vi "PM100D2&D3 SCPI Example.vi"() -> ()   [LabVIEW 2015]
uses:
  <vilib>/ErrorRing/Error Ring.xnode
  <vilib>/Utility/error.llb/Error Cluster From Error Code.vi
panel:
  in  "stop":bool
  out "ARR LEN":i32
  out "rate":dbl format="%#.2f"
  out "count":i32
  out "time":u32
  out "error out":errorcluster
  in  "Tab Control":T1(tab)
  out "Chart":dbl(graph)
  in  "Scope Mode Array Length":i32=100
  out "Scope Mode Array [timestamp(us), power(W)]":cluster{u32, sgl}[](array[cluster])
  in  "Burst Mode Array Length":i32=100
  out "Burst Mode Array [timestamp(us), power(W)]":cluster{u32, sgl}[](array[cluster])
  out "Product Info":string
  # "Average Sampling Rate (Samples/s)"
  # "(range is 1 to 100)"
  # "I/O ports are 5 V TTL tolerant. The start of measurement is triggered on the rising edge of the TTL signal. In this example, the GPIO1 is configured as IALT."
  # "(range is 1 to 100)"
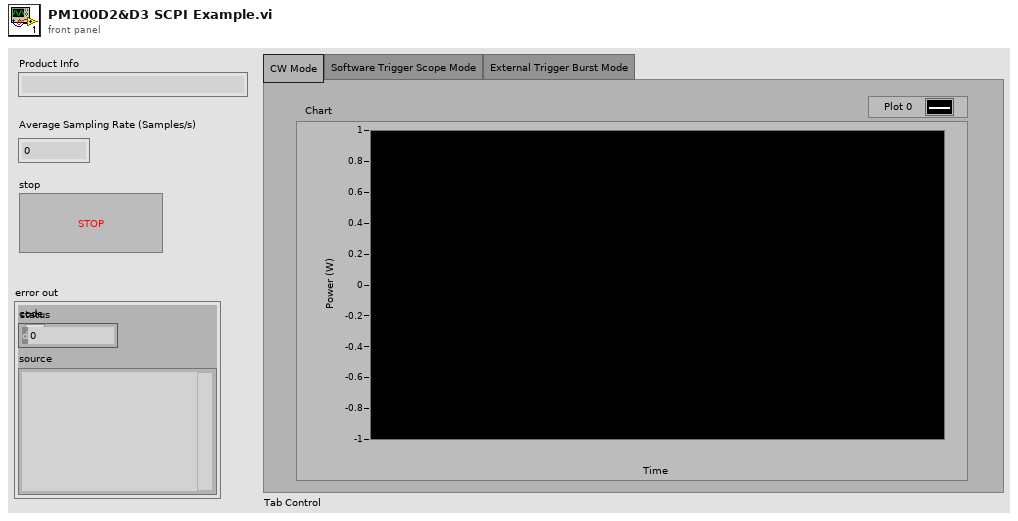
[diagram p1: front panel]
types:
  T1 = enum32{"CW Mode", "Software Trigger Scope Mode", "External Trigger Burst Mode"}
  T2 = enum16{"big-endian, network order", "native, host order", "little-endian"}
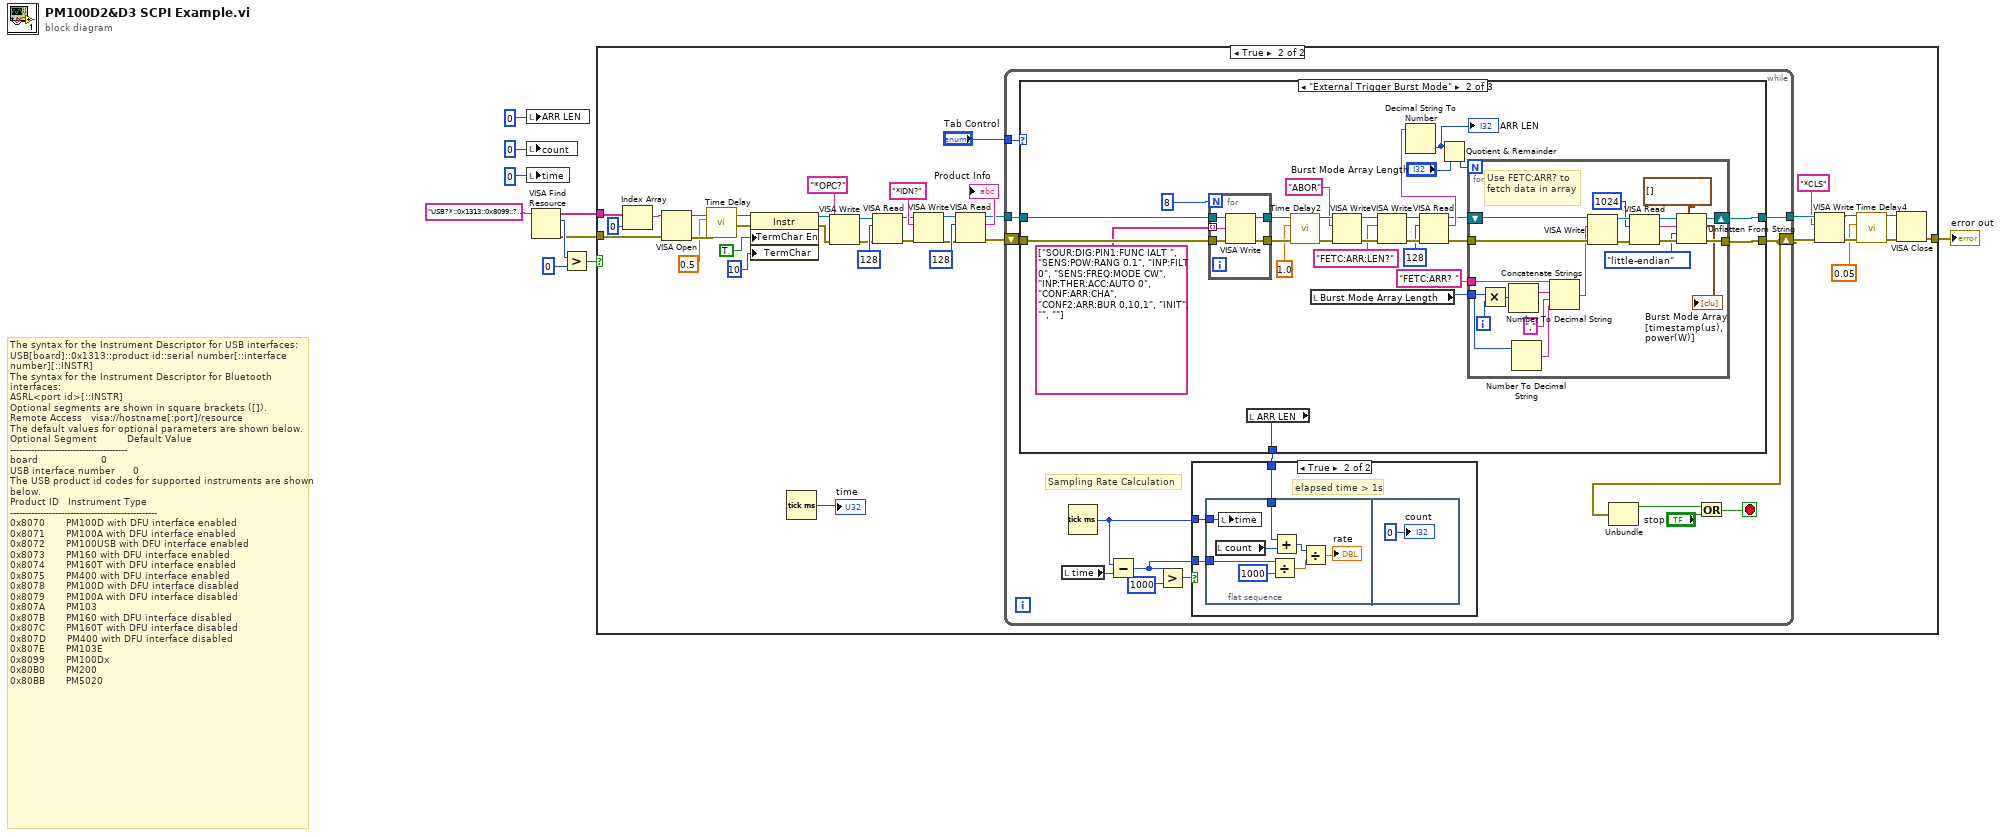
[diagram p0: block diagram]
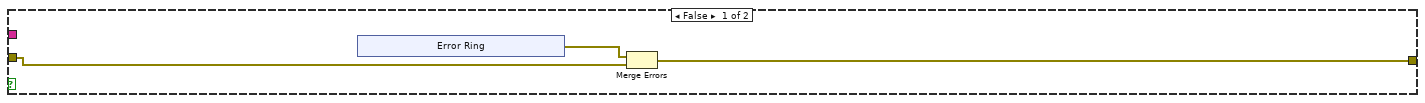
[diagram p2: hidden frame]
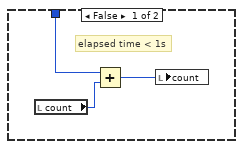
[diagram p3: hidden frame]
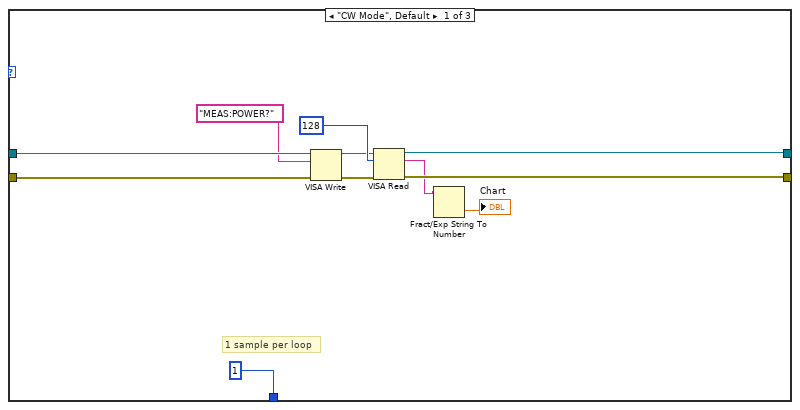
[diagram p4: hidden frame]
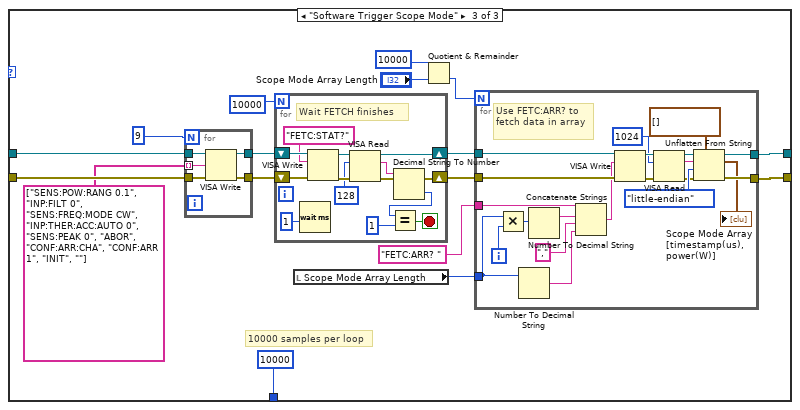
[diagram p5: hidden frame]
diagram:
  # "The syntax for the Instrument Descriptor for USB interfaces:\nUSB[board]::0x1313::product id::serial number[::interface number][::INSTR]\nThe syntax for the Instrument Descriptor for Bluetooth interfaces:\nASRL<port id>[::INSTR]\nOptional segments are shown in square brackets ([]).\nRemote Access   visa://hostname[:port]/resource\nThe default values for optional parameters are shown below.\nOptional Segment          Default Value\n---------------------------------------\nboard                     0\nUSB interface number      0\nThe USB product id codes for supported instruments are shown below.\nProduct ID   Instrument Type\n-------------------------------------------------\n0x8070       PM100D with DFU interface enabled\n0x8071       PM100A with DFU interface enabled\n0x8072       PM100USB with DFU interface enabled\n0x8073       PM160 with DFU interface enabled\n0x8074       PM160T with DFU interface enabled\n0x8075       PM400 with DFU interface enabled\n0x8078       PM100D with DFU interface disabled\n0x8079       PM100A with DFU interface disabled\n0x807A       PM103\n0x807B       PM160 with DFU interface disabled\n0x807C       PM160T with DFU interface disabled\n0x807D       PM400 with DFU interface disabled\n0x807E       PM103E\n0x8099       PM100Dx\n0x80B0       PM200\n0x80BB       PM5020"
  n1 = local write "ARR LEN"(0 ("ARR LEN")) -> ()
  n2 = local write "count"(0 ("loopCount")) -> ()
  n3 = local write "time"(u32 0 ("time")) -> ()
  n4 = VISA Find Resource(11:"USB?*::0x1313::0x8099::?*::INSTR" ("expression (\"?*\")")) -> (0:w4:errorcluster, 2:w9:u32, 3:w6:string[])  [unwired: 2 in]
  n5 = Greater?(x=w9, y=u32 0) -> (0:w7:bool)
  n6 = case shown="True" w7 {
    tunnel: w6 -> [_ w53]
    tunnel: [w13 w26] -> w5
    tunnel: w4 -> [w12 w38]
    frame False {
      n7 = xnode "Error Ring"() -> ("error out"=w11:errorcluster)
      n8 = Merge Errors(w11, w12) -> (w13:errorcluster)
    }
    frame True {
      n9 = Index Array(array=w53, index=0) -> (element=w39:string)
      n10 = VISA Open(error in (no error)=w38, VISA resource name=w39) -> (VISA resource name=w45:refnum<visa-resource-name>, error out=w48:errorcluster)  [unwired: 3 in]
      n11 = call "Time Delay"("error in (no error)"=w48, "Delay Time (s)"=0.5) -> ("error out"=w46:errorcluster)  [unwired: 9 in]
      n12 = property class="Instr"(reference=w45, error in=w46, "TermChar En"=TRUE ("Message Based Settings:Termination Character Enable"), "TermChar"=u8 10 ("Message Based Settings:Termination Character")) -> (reference out=w22:refnum<visa-resource-name>, error out=w21:errorcluster)
      n13 = Tick Count (ms)() -> (millisecond timer value=→"time":u32)
      n14 = VISA Write(VISA resource name=w22, write buffer="*OPC?", error in (no error)=w21) -> (VISA resource name out=w34:refnum<visa-resource-name>, error out=w19:errorcluster)  [unwired: 1 out]
      n15 = VISA Read(VISA resource name=w34, byte count=u32 128, error in (no error)=w19) -> (VISA resource name out=w33:refnum<visa-resource-name>, error out=w36:errorcluster)  [unwired: 2 out]
      n16 = VISA Write(VISA resource name=w33, write buffer="*IDN?", error in (no error)=w36) -> (VISA resource name out=w50:refnum<visa-resource-name>, error out=w25:errorcluster)  [unwired: 1 out]
      n17 = VISA Read(VISA resource name=w50, byte count=u32 128, error in (no error)=w25) -> (VISA resource name out=w42:refnum<visa-resource-name>, read buffer=→"Product Info":string, error out=w41:errorcluster)  [unwired: 1 out]
      n18 = while {
        tunnel: [w67] -> w31
        tunnel: w42 -> [w66]
        tunnel: "Tab Control" -> [w64]
        shift-right: [w56] -> w32
        shift-left: w41 -> [w65]
        stop <- w54 stop-if-true
        # "Sampling Rate Calculation"
        n19 = case shown="\"External Trigger Burst Mode\"" w64 {
          tunnel: [w90 w117 w159] -> w67
          tunnel: w66 -> [w92 w118 w160]
          tunnel: [w89 w119 w161] -> w56
          tunnel: w65 -> [w91 w116 w146]
          tunnel: [1 w115 10000 ("x")] -> w61
          frame "CW Mode", Default {
            # "1 sample per loop"
            n20 = VISA Write(VISA resource name=w92, write buffer="MEAS:POWER?", error in (no error)=w91) -> (VISA resource name out=w84:refnum<visa-resource-name>, error out=w83:errorcluster)  [unwired: 1 out]
            n21 = VISA Read(VISA resource name=w84, byte count=u32 128, error in (no error)=w83) -> (VISA resource name out=w90:refnum<visa-resource-name>, read buffer=w87:string, error out=w89:errorcluster)  [unwired: 1 out]
            n22 = Fract/Exp String To Number(string=w87) -> (number=→"Chart":dbl)  [unwired: 3 in, 1 out]
          }
          frame "External Trigger Burst Mode" {
            n23 = for {
              N: 8 -> [_]
              tunnel: string[] ["SOUR:DIG:PIN1:FUNC IALT ", "SENS:POW:RANG 0.1", "INP:FILT 0", "SENS:FREQ:MODE CW", "INP:THER:ACC:AUTO 0", "CONF:ARR:CHA", "CONF2:ARR:BUR 0,10,1", "INIT", "", ""] -> [w142] mode=indexing
              tunnel: w116 -> [w144]
              tunnel: w118 -> [w143]
              tunnel: [w141] -> w112
              tunnel: [w140] -> w109
              n24 = VISA Write(VISA resource name=w143, write buffer=w142, error in (no error)=w144) -> (VISA resource name out=w140:refnum<visa-resource-name>, error out=w141:errorcluster)  [unwired: 1 out]
            }
            n25 = local read "ARR LEN"() -> (w115:i32)
            n26 = call "Time Delay2"("error in (no error)"=w112, "Delay Time (s)"=1.0) -> ("error out"=w110:errorcluster)  [unwired: 9 in]
            n27 = local read "Burst Mode Array Length"() -> (w94:i32)
            n28 = VISA Write(VISA resource name=w109, write buffer="ABOR", error in (no error)=w110) -> (VISA resource name out=w106:refnum<visa-resource-name>, error out=w107:errorcluster)  [unwired: 1 out]
            n29 = VISA Write(VISA resource name=w106, write buffer="FETC:ARR:LEN?", error in (no error)=w107) -> (VISA resource name out=w103:refnum<visa-resource-name>, error out=w104:errorcluster)  [unwired: 1 out]
            n30 = VISA Read(VISA resource name=w103, byte count=u32 128, error in (no error)=w104) -> (VISA resource name out=w99:refnum<visa-resource-name>, read buffer=w101:string, error out=w100:errorcluster)  [unwired: 1 out]
            n31 = Decimal String To Number(string=w101) -> (number=w97:i32)  [unwired: 2 in, 1 out]
            "ARR LEN" <- w97
            n32 = Quotient & Remainder(x=w97, y="Burst Mode Array Length") -> (floor(x/y)=w95:i32)  [unwired: 1 out]
            n33 = for {
              N: w95 -> [_]
              tunnel: w100 -> [w139]
              tunnel: "FETC:ARR? " ("write buffer") -> [w129]
              tunnel: [w126] -> w119
              tunnel: w94 -> [w121]
              shift-right: [w134] -> w117
              shift-left: w99 -> [w137]
              i -> [w120]
              # "Use FETC:ARR? to fetch data in array"
              n34 = Multiply(x=w121, y=w120) -> (x*y=w131:i32)
              n35 = Number To Decimal String(number=w131) -> (decimal integer string=w133:string)  [unwired: 1 in]
              n36 = Number To Decimal String(number=w121) -> (decimal integer string=w130:string)  [unwired: 1 in]
              n37 = Concatenate Strings(w129, w133, "," ("string"), w130) -> (w128:string)
              n38 = VISA Write(VISA resource name=w137, write buffer=w128, error in (no error)=w139) -> (VISA resource name out=w136:refnum<visa-resource-name>, error out=w138:errorcluster)  [unwired: 1 out]
              n39 = VISA Read(VISA resource name=w136, byte count=u32 1024, error in (no error)=w138) -> (VISA resource name out=w134:refnum<visa-resource-name>, read buffer=w123:string, error out=w127:errorcluster)  [unwired: 1 out]
              n40 = Unflatten From String(type=cluster{u32, sgl}[] [], binary string=w123, byte order (0:big-endian, network order)=T2."little-endian", error in (no error)=w127) -> (value=→"Burst Mode Array [timestamp(us), power(W)]":cluster{u32, sgl}[], error out=w126:errorcluster)  [unwired: 1 in, 1 out]
            }
          }
          frame "Software Trigger Scope Mode" {
            # "10000 samples per loop"
            n41 = for {
              N: 9 -> [_]
              tunnel: w146 -> [w199]
              tunnel: w160 -> [w198]
              tunnel: [w197] -> w152
              tunnel: [w196] -> w156
              tunnel: string[] ["SENS:POW:RANG 0.1", "INP:FILT 0", "SENS:FREQ:MODE CW", "INP:THER:ACC:AUTO 0", "SENS:PEAK 0", "ABOR", "CONF:ARR:CHA", "CONF:ARR 1", "INIT", ""] -> [w195] mode=indexing
              n42 = VISA Write(VISA resource name=w198, write buffer=w195, error in (no error)=w199) -> (VISA resource name out=w196:refnum<visa-resource-name>, error out=w197:errorcluster)  [unwired: 1 out]
            }
            n43 = for {
              N: 10000 -> [_]
              shift-right: [w169] -> w154
              shift-left: w156 -> [w174]
              shift-right: [w168] -> w153
              shift-left: w152 -> [w172]
              stop <- w163 stop-if-true
              # "Wait FETCH finishes"
              n44 = Wait (ms)(milliseconds to wait=u32 1) -> ()  [unwired: 1 out]
              n45 = VISA Write(VISA resource name=w174, write buffer="FETC:STAT?", error in (no error)=w172) -> (VISA resource name out=w170:refnum<visa-resource-name>, error out=w171:errorcluster)  [unwired: 1 out]
              n46 = VISA Read(VISA resource name=w170, byte count=u32 128, error in (no error)=w171) -> (VISA resource name out=w169:refnum<visa-resource-name>, read buffer=w166:string, error out=w168:errorcluster)  [unwired: 1 out]
              n47 = Decimal String To Number(string=w166) -> (number=w165:i32)  [unwired: 2 in, 1 out]
              n48 = Equal?(x=w165, y=1) -> (x = y?=w163:bool)
            }
            n49 = local read "Scope Mode Array Length"() -> (w147:i32)
            n50 = Quotient & Remainder(x=10000, y="Scope Mode Array Length") -> (floor(x/y)=w150:i32)  [unwired: 1 out]
            n51 = for {
              N: w150 -> [_]
              tunnel: w153 -> [w194]
              tunnel: w154 -> [w192]
              tunnel: "FETC:ARR? " ("write buffer") -> [w190]
              tunnel: [w186] -> w159
              tunnel: [w181] -> w161
              tunnel: w147 -> [w177]
              i -> [w179]
              # "Use FETC:ARR? to fetch data in array"
              n52 = Multiply(x=w177, y=w179) -> (x*y=w180:i32)
              n53 = Number To Decimal String(number=w177) -> (decimal integer string=w178:string)  [unwired: 1 in]
              n54 = Number To Decimal String(number=w180) -> (decimal integer string=w189:string)  [unwired: 1 in]
              n55 = Concatenate Strings(w190, w189, "," ("string"), w178) -> (w188:string)
              n56 = VISA Write(VISA resource name=w192, write buffer=w188, error in (no error)=w194) -> (VISA resource name out=w191:refnum<visa-resource-name>, error out=w193:errorcluster)  [unwired: 1 out]
              n57 = VISA Read(VISA resource name=w191, byte count=u32 1024, error in (no error)=w193) -> (VISA resource name out=w186:refnum<visa-resource-name>, read buffer=w184:string, error out=w182:errorcluster)  [unwired: 1 out]
              n58 = Unflatten From String(type=cluster{u32, sgl}[] [], binary string=w184, byte order (0:big-endian, network order)=T2."little-endian", error in (no error)=w182) -> (value=→"Scope Mode Array [timestamp(us), power(W)]":cluster{u32, sgl}[], error out=w181:errorcluster)  [unwired: 1 in, 1 out]
            }
          }
        }
        n59 = local read "time"() -> (w60:u32)
        n60 = Tick Count (ms)() -> (millisecond timer value=w62:u32)
        n61 = Subtract(x=w62, y=w60) -> (x-y=w59:u32)
        n62 = Greater?(x=w59, y=u32 1000) -> (0:w55:bool)
        n63 = case shown="True" w55 {
          tunnel: w62 -> [_ w73]
          tunnel: w61 -> [w69 w71]
          tunnel: w59 -> [_ w72]
          frame False {
            # "elapsed time < 1s"
            n64 = local read "count"() -> (w70:i32)
            n65 = Add(x=w69, y=w70) -> (x+y=w68:i32)
            n66 = local write "count"(w68) -> ()
          }
          frame True {
            # "elapsed time > 1s"
            n67 = flat-sequence {
              tunnel: w73 -> [w81]
              tunnel: w72 -> [w78]
              tunnel: w71 -> [w74]
              frame #0 {
                n68 = local read "count"() -> (w75:i32)
                n69 = local write "time"(w81) -> ()
                n70 = Divide(x=w78, y=u32 1000) -> (x/y=w79:dbl)
                n71 = Add(x=w74, y=w75) -> (x+y=w76:i32)
                n72 = Divide(x=w76, y=w79) -> (x/y=→"rate":dbl)
              }
              frame #1 {
                "count" <- 0 ("count")
              }
            }
          }
        }
        n73 = Unbundle(w56) -> ("status"=w57:bool)  [unwired: 2 out]
        n74 = Or(x=w57, y="stop") -> (x .or. y?=w54:bool)
      }
      n75 = VISA Write(VISA resource name=w31, write buffer="*CLS", error in (no error)=w32) -> (VISA resource name out=w30:refnum<visa-resource-name>, error out=w28:errorcluster)  [unwired: 1 out]
      n76 = call "Time Delay4"("error in (no error)"=w28, "Delay Time (s)"=0.05) -> ("error out"=w27:errorcluster)  [unwired: 9 in]
      n77 = VISA Close(VISA resource name=w30, error in (no error)=w27) -> (error out=w26:errorcluster)
    }
  }
  "error out" <- w5
